vi "SSL UDP Receiver.vi"(10 "SSL UDP Receiver 2":refnum<vi>, 11 "SSL UDP Receiver":T1={"Port:"=10020, "Server IP:"="224.5.23.2", "Local IP:"="224.5.23.2", "RX"=FALSE}) -> (0 "error out":errorcluster, 3 "Channel out":T2)   [LabVIEW 2017]
uses:
  <extravilib>/ChannelInstances/Lossy Stream-a[.](u8)/)Channel.ctl
  Control/SSL UDP Address.ctl
  <extravilib>/ChannelInstances/Lossy Stream-a[.](u8)/Write With Abort.vi
  <extravilib>/ChannelInstances/Lossy Stream-a[.](u8)/Endpoint.vi
  <extravilib>/ChannelInstances/Lossy Stream-a[.](u8)/)Channel.vi
  <vilib>/Utility/tcp.llb/UDP Multicast Read-Only Open.vi
  <extravilib>/ChannelInstances/Lossy Stream-a[.](u8).lvlib
panel:
  out "error out 3":errorcluster
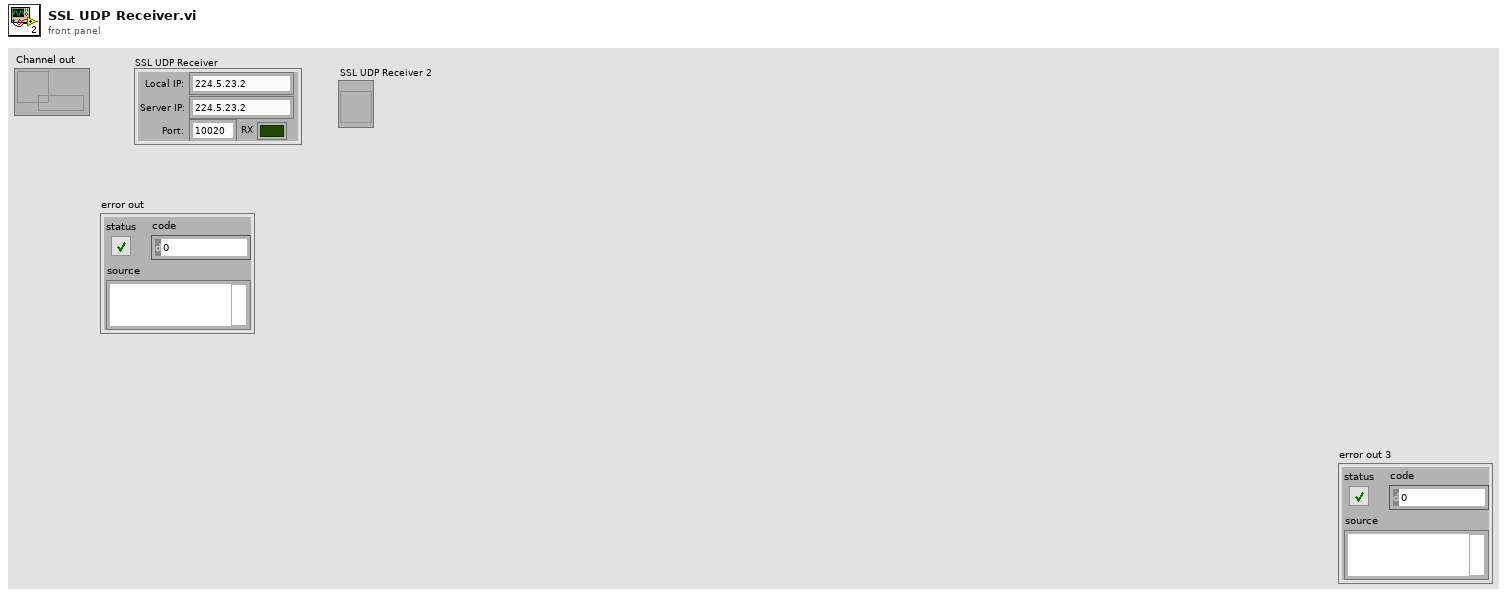
[diagram p1: front panel]
types:
  T1 = typedef "SSL UDP Address.ctl" = cluster{"Port:":u16, "Server IP:":string, "Local IP:":string, "RX":bool}
  T2 = typedef "Lossy Stream-a[.](u8).lvlib/)Channel.ctl" = refnum<queue>
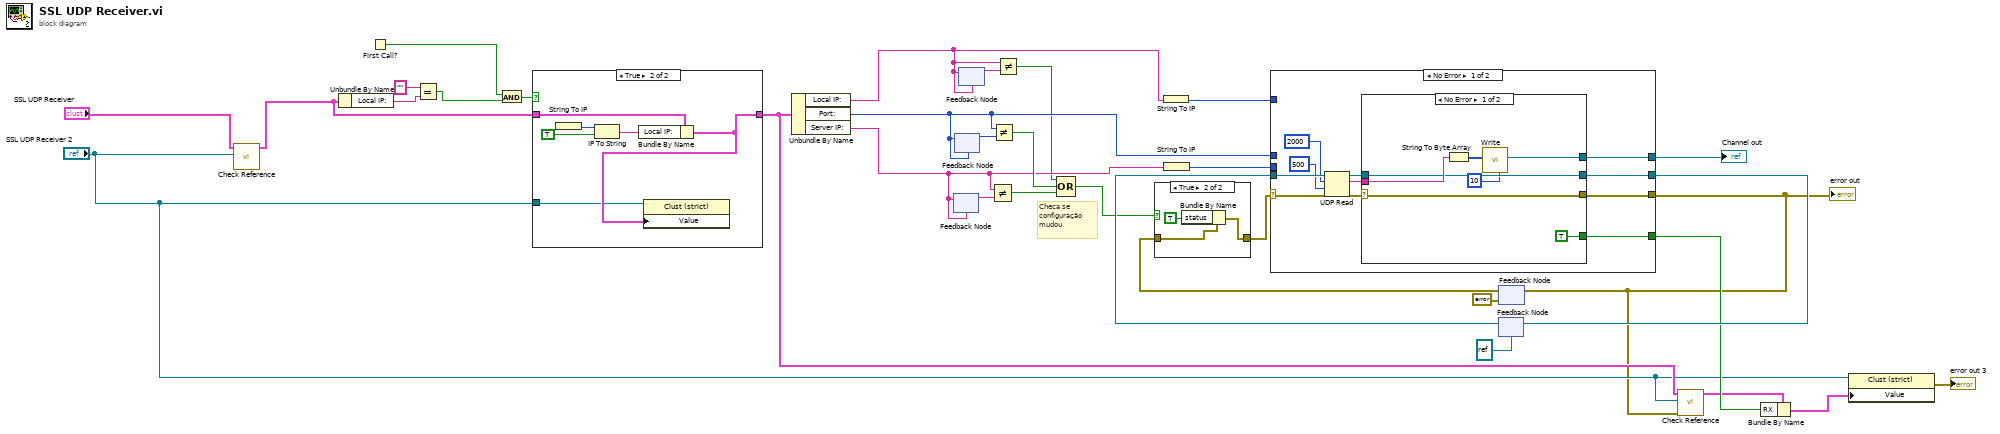
[diagram p0: block diagram]
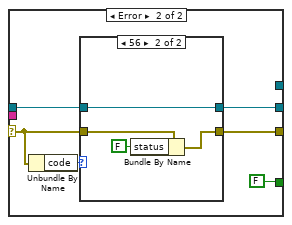
[diagram p4: hidden frame]
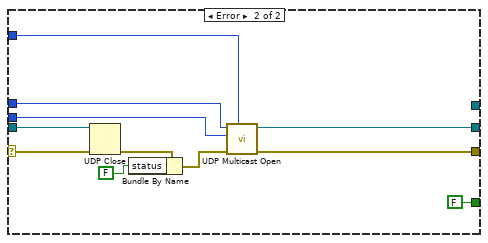
[diagram p6: hidden frame]
diagram:
  # "Checa se \nconfiguração\nmudou"
  n1 = call "Check Reference.vi"("Cluster in"="SSL UDP Receiver 2", "SSL UDP Receiver 3"="SSL UDP Receiver") -> ("SSL UDP Receiver"=w12:T1)  [unwired: 8 in, 1 out]
  n2 = Unbundle By Name(w12) -> ("Local IP:"=w11:string)
  n3 = First Call?() -> (First Call?: T/F=w14:bool)
  n4 = Equal?(x="", y=w11) -> (x = y?=w9:bool)
  n5 = And(x=w14, y=w9) -> (x .and. y?=w13:bool)
  n6 = case shown="True" w13 {
    tunnel: [w34 w36] -> w4
    tunnel: w12 -> [w34 w40]
    tunnel: "SSL UDP Receiver 2" -> [_ w35]
    frame False {
    }
    frame True {
      n7 = String To IP() -> (0:w38:u32)  [unwired: 1 in]
      n8 = IP To String(1:TRUE ("dot notation? (F)"), 2:w38) -> (0:w39:string)
      n9 = Bundle By Name(cluster=w40, "Local IP:"=w39) -> (w36:T1)
      n10 = property on="Property Node" class="Clust (strict)"(reference=w35, "Value"=w36) -> ()  [unwired: 1 in, 2 out]
    }
  }
  n11 = Unbundle By Name(w4) -> ("Local IP:"=w16:string, "Port:"=w20:u16, "Server IP:"=w19:string)
  n12 = feedback-in #1(w19) -> ()
  n13 = feedback #1(w19) -> (w25:string)
  n14 = feedback #2(w20) -> (w23:u16)
  n15 = feedback-in #2(w20) -> ()
  n16 = feedback #3(w16) -> (w18:string)
  n17 = feedback-in #3(w16) -> ()
  n18 = Not Equal?(x=w19, y=w25) -> (x != y?=w24:bool)
  n19 = Not Equal?(x=w20, y=w23) -> (x != y?=w22:bool)
  n20 = Not Equal?(x=w16, y=w18) -> (x != y?=w17:bool)
  n21 = Compound Arithmetic op=OR(w17, w22, w24) -> (w21:bool)
  n22 = String To IP(1:w16) -> (0:w15:u32)
  n23 = String To IP(1:w19) -> (0:w30:u32)
  n24 = feedback #4(refnum<k16> refnum ("connection ID")) -> (w31:refnum<k16>)
  n25 = feedback #5(errorcluster {"status"=TRUE, "code"=0, "source"=""} ("error out")) -> (w27:errorcluster)
  n26 = case shown="True" w21 {
    tunnel: w27 -> [w41 w43]
    tunnel: [w41 w42] -> w26
    frame False {
    }
    frame True {
      n27 = Bundle By Name(cluster=w43, "status"=TRUE) -> (w42:errorcluster)
    }
  }
  n28 = case shown="No Error" w26 {
    selector: w26 -> [w45 w76]
    tunnel: w31 -> [w55 w82]
    tunnel: [w54 _] -> w33
    tunnel: [w53 w84] -> w1
    tunnel: [w52 w85] -> w32
    tunnel: w20 -> [_ w83]
    tunnel: w30 -> [_ w81]
    tunnel: [w46 FALSE] -> w7
    tunnel: w15 -> [_ w75]
    frame No Error {
      n29 = UDP Read(connection ID=w55, max size (548)=2000, timeout ms (25000)=500, 8:w45) -> (data out=w49:string, error out=w47:errorcluster, 3:w48:refnum<k16>)  [unwired: 2 out]
      n30 = case shown="No Error" w47 {
        selector: w47 -> [w57 w63]
        tunnel: [w59 _] -> w54
        tunnel: w49 -> [w62 _]
        tunnel: [w57 w65] -> w53
        tunnel: [w61 w66] -> w52
        tunnel: w48 -> [w61 w67]
        tunnel: [TRUE FALSE] -> w46
        frame No Error {
          n31 = String To Byte Array(string=w62) -> (unsigned byte array=w60:u8[])
          n32 = call <extravilib>:"Write.vi"("size (1)"=10, "element"=w60) -> ("channel"=w59:T2)  [unwired: 7 in, 2 out]
        }
        frame Error {
          n33 = Unbundle By Name(w63) -> ("code"=w68:i32)
          n34 = case shown="56" w68 {
            tunnel: w63 -> [w70 w74]
            tunnel: [w70 w72] -> w65
            tunnel: w67 -> [w69 w71]
            tunnel: [w69 w71] -> w66
            frame Default {
            }
            frame 56 {
              n35 = Bundle By Name(cluster=w74, "status"=FALSE) -> (w72:errorcluster)
            }
          }
        }
      }
    }
    frame Error {
      n36 = UDP Close(connection ID=w82, 8:w76) -> (error out=w79:errorcluster)  [unwired: 1 out]
      n37 = Bundle By Name(cluster=w79, "status"=FALSE) -> (w77:errorcluster)
      n38 = call-poly <vilib>:"UDP Multicast Open.vi"("net address"=w75, "error in (no error)"=w77, "multicast addr"=w81, "port"=w83) -> ("error out"=w84:errorcluster, "connection ID"=w85:refnum<k16>)  [unwired: 5 in, 1 out]
    }
  }
  "error out" <- w1
  "Channel out" <- w33
  n39 = feedback-in #4(w32) -> ()
  n40 = feedback-in #5(w1) -> ()
  n41 = call "Check Reference.vi"("error in (no error)"=w1, "Cluster in"="SSL UDP Receiver 2", "SSL UDP Receiver 3"=w4) -> ("SSL UDP Receiver"=w2:T1)  [unwired: 7 in, 1 out]
  n42 = Bundle By Name(cluster=w2, "RX"=w7) -> (w6:T1)
  n43 = property on="Property Node" class="Clust (strict)"(reference="SSL UDP Receiver 2", "Value"=w6) -> (error out=→"error out 3":errorcluster)  [unwired: 1 in, 1 out]
